vi "PID-DruckRegler erweitert.vi"(0 "Sollwert":sgl, 1 "Regler EIN":bool=TRUE, 2 "Regler Interne Werte":sgl[](array[numeric]), 5 "Istwert":sgl, 7 "PID-Parameter":T2 {"Regler Toleranz -" format="%_2f"; "Regler Toleranz +" format="%_2f"; "D-Anteil" format="%_2f"; "I-Anteil" format="%_2f"; "P-Anteil" format="%_2f"}, 9 "output range":cluster{"output high":sgl, "output low":sgl}={"output high"=100.0, "output low"=-100.0} {"output low" format="%.2f"; "output high" format="%.2f"}, 11 "Werte vorgeben":bool=TRUE, 12 "Regler Toleranz verwenden?":bool=TRUE) -> (3 "Regler Interne Werte":T1, 4 "Interne Werte speichern":bool, 6 "Im Bereich":bool, 8 "Output":sgl)   [LabVIEW 2020, in "Regler.lvlib" / "Druckregler.lvlib"]
uses:
  Druckregler.lvlib
  Regler Interne Werte.ctl
  Regler Werte erzwingen.ctl
  <vilib>/addons/control/pid/pid.llb/PID Control Input Filter (DBL).vi
  <vilib>/addons/control/pid/NI_PID_pid.lvlib
  Allgemein/Allgemein.lvlib
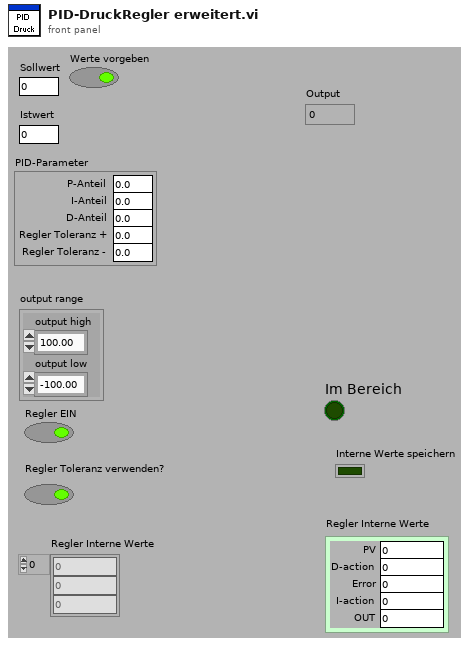
[diagram p1: front panel]
types:
  T1 = typedef "Regler.lvlib/Druckregler.lvlib/Regler Interne Werte.ctl" = cluster{"PV":sgl, "D-action":sgl, "Error":sgl, "I-action":sgl, "OUT":sgl}
  T2 = cluster{"P-Anteil":sgl, "I-Anteil":sgl, "D-Anteil":sgl, "Regler Toleranz +":sgl, "Regler Toleranz -":sgl}
  T3 = typedef "Regler.lvlib/Druckregler.lvlib/Regler Werte erzwingen.ctl" = enum16{"normal", "erzwingen"}
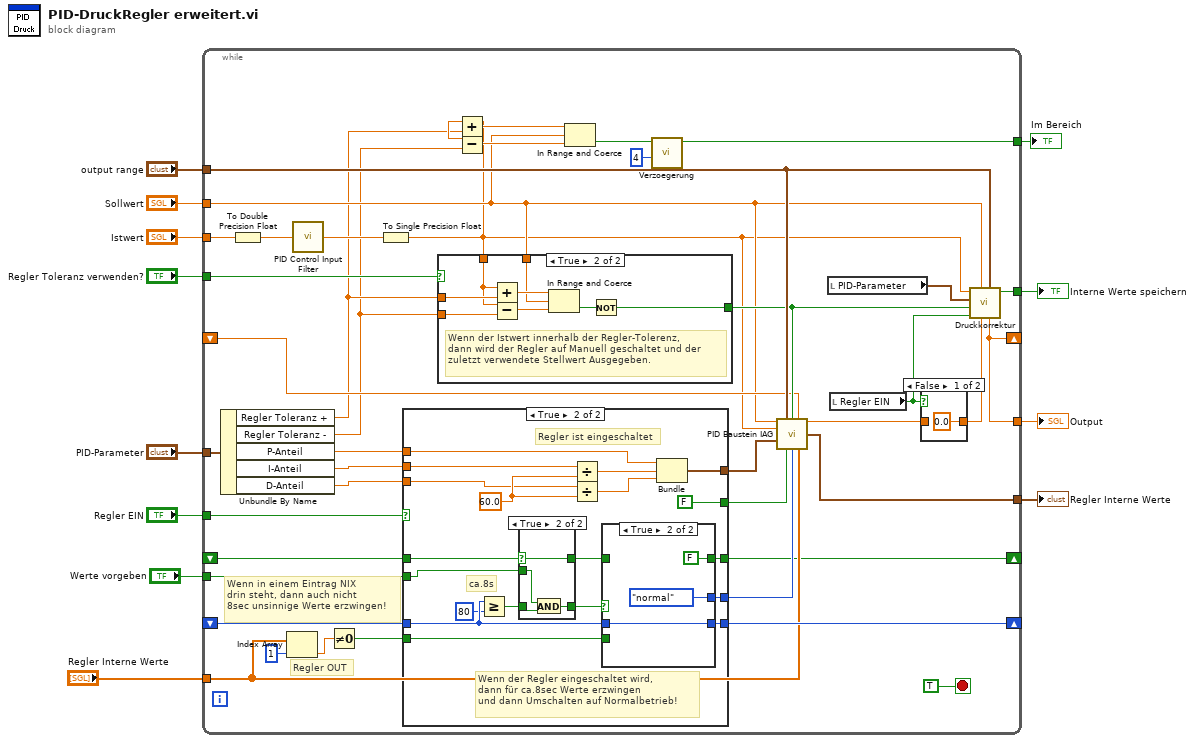
[diagram p0: block diagram]
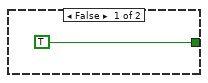
[diagram p2: hidden frame]
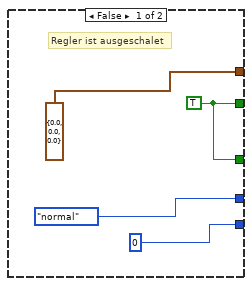
[diagram p4: hidden frame]
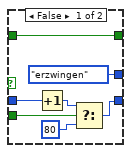
[diagram p6: hidden frame]
diagram:
  n1 = while {
    tunnel: "PID-Parameter" -> [w53]
    tunnel: "Regler EIN" -> [w49]
    tunnel: "Regler Toleranz verwenden?" -> [w45]
    tunnel: "output range" -> [w44]
    tunnel: [w29] -> w8
    tunnel: "Sollwert" -> [w22]
    tunnel: "Istwert" -> [w41]
    tunnel: [w36] -> w5
    tunnel: "Regler Interne Werte" -> [w27]
    shift-right: [w34] -> _
    shift-left: _ -> [w33]
    tunnel: [w31] -> w4
    shift-right: [w29] -> _
    shift-left: _ -> [w28]
    tunnel: [w17] -> w2
    shift-right: [w16] -> _
    shift-left: _ -> [w15]
    tunnel: "Werte vorgeben" -> [w14]
    stop <- TRUE stop-if-true
    # "Regler OUT"
    # "Wenn in einem Eintrag NIX\ndrin steht, dann auch nicht \n8sec unsinnige Werte erzwingen!"
    n2 = Unbundle By Name(w53) -> ("Regler Toleranz +"=w20:sgl, "Regler Toleranz -"=w19:sgl, "P-Anteil"=w52:sgl, "I-Anteil"=w51:sgl, "D-Anteil"=w50:sgl)
    n3 = To Double Precision Float(number=w41) -> (double precision float=w40:dbl)
    n4 = Index Array(array=w27, index=1 ("Index")) -> (element=w25:sgl)
    n5 = call-poly <vilib>:"PID Control Input Filter.vi"("input"=w40) -> ("output"=w39:dbl)  [unwired: 4 in]
    n6 = Not Equal To 0?(x=w25) -> (x != 0?=w30:bool)
    n7 = To Single Precision Float(number=w39) -> (single precision float=w21:sgl)
    n8 = case shown="True" w49 {
      tunnel: [cluster{"P-Anteil":sgl, sgl, sgl} {"P-Anteil"=0.0, 0.0, 0.0} w80] -> w48
      tunnel: w52 -> [_ w81]
      tunnel: w51 -> [_ w85]
      tunnel: w50 -> [_ w84]
      tunnel: [w65 FALSE] -> w47
      tunnel: [u16 0 w79] -> w34
      tunnel: w33 -> [_ w78]
      tunnel: [Regler_Werte_erzwingen."normal" ("Regler erzwingen") w76] -> w32
      tunnel: w30 -> [_ w75]
      tunnel: [w65 w70] -> w16
      tunnel: w15 -> [_ w72]
      tunnel: w14 -> [_ w69]
      frame False {
        w65 = TRUE
        # "Regler ist ausgeschalet"
      }
      frame True {
        w86 = sgl 60.0 ("y")
        # "Wenn der Regler eingeschaltet wird, \ndann für ca.8sec Werte erzwingen \nund dann Umschalten auf Normalbetrieb!"
        # "ca.8s"
        # "Regler ist eingeschaltet"
        n9 = Greater Or Equal?(x=w78, y=u16 80) -> (x >= y?=w73:bool)
        n10 = case shown="True" w72 {
          selector: w72 -> [w88 w91]
          tunnel: [w89 w93] -> w74
          tunnel: w73 -> [w89 w92]
          tunnel: [w88 w91] -> w71
          tunnel: w69 -> [_ w90]
          frame False {
          }
          frame True {
            n11 = And(x=w90, y=w92) -> (x .and. y?=w93:bool)
          }
        }
        n12 = Divide(x=w85, y=w86) -> (x/y=w83:sgl)
        n13 = Divide(x=w84, y=w86) -> (x/y=w82:sgl)
        n14 = case shown="True" w74 {
          tunnel: w78 -> [w100 w103]
          tunnel: [w96 w103] -> w79
          tunnel: [Regler_Werte_erzwingen."erzwingen" ("Regler erzwingen") Regler_Werte_erzwingen."normal" ("Regler erzwingen")] -> w76
          tunnel: w75 -> [w98 _]
          tunnel: w71 -> [w94 _]
          tunnel: [w94 FALSE] -> w70
          frame False {
            n15 = Increment(x=w100) -> (x+1=w97:u16)
            n16 = Select(t=w97, s=w98, f=u16 80) -> (s? t:f=w96:u16)
          }
          frame True {
          }
        }
        n17 = Bundle("P-Anteil"=w81, w83, w82) -> (w80:cluster{"P-Anteil":sgl, sgl, sgl})  [unwired: 1 in]
      }
    }
    n18 = case shown="True" w45 {
      tunnel: [TRUE w61] -> w43
      tunnel: w21 -> [_ w56]
      tunnel: w20 -> [_ w60]
      tunnel: w19 -> [_ w59]
      tunnel: w22 -> [_ w55]
      frame False {
      }
      frame True {
        # "Wenn der Istwert innerhalb der Regler-Tolerenz,\ndann wird der Regler auf Manuell geschaltet und der \nzuletzt verwendete Stellwert Ausgegeben."
        n19 = Add(x=w56, y=w60) -> (x+y=w58:sgl)
        n20 = Subtract(x=w56, y=w59) -> (x-y=w57:sgl)
        n21 = In Range and Coerce(upper limit=w58, x=w55, lower limit=w57) -> (In Range?=w62:bool)  [unwired: 1 out]
        n22 = Not(x=w62) -> (.not. x?=w61:bool)
      }
    }
    n23 = Add(x=w21, y=w20) -> (x+y=w23:sgl)
    n24 = Subtract(x=w21, y=w19) -> (x-y=w24:sgl)
    n25 = In Range and Coerce(upper limit=w23, x=w22, lower limit=w24) -> (In Range?=w13:bool)  [unwired: 1 out]
    n26 = call "Verzoegerung.vi"("sec"=u16 4, "Startsignal"=w13) -> ("Zeit abgelaufen?"=w17:bool)  [unwired: 8 in, 1 out]
    n27 = call "PID Baustein IAG.vi"("setpoint"=w22, "output range"=w44, "auto? (T)"=w43, "manual control"=w28, "process variable"=w21, "PID gains"=w48, "reinitialize? (F)"=w47, "Regler erzwingen"=w32, "Regler Interne Werte"=w27) -> ("output"=w46:sgl, "Regler Werte"=w36:T1)  [unwired: 4 in, 1 out]
    n28 = local read "PID-Parameter"() -> (w38:T2)
    n29 = local read "Regler EIN"() -> (w37:bool)
    n30 = case shown="False" w37 {
      tunnel: [sgl 0.0 w64] -> w42
      tunnel: w46 -> [_ w64]
      frame False {
      }
      frame True {
      }
    }
    n31 = call "Druckkorrektur.vi"("output range"=w44, "Output"=w42, "Sollwert"=w22, "Regler EIN"=w37, "Auto?"=w43, "PID-Parameter"=w38, "Istwert"=w21) -> ("Interne Werte speichern"=w31:bool, "Output"=w29:sgl)  [unwired: 3 in]
  }
  "Output" <- w8
  "Regler Interne Werte" <- w5
  "Interne Werte speichern" <- w4
  "Im Bereich" <- w2
